vi "GetOutput.vi"(4 "error in":errorcluster, 5 "connection ID":refnum<k5>) -> (0 "Output":string, 1 "error out":errorcluster, 2 "connection ID out":refnum<k5>, 3 "Answer":bool)   [LabVIEW 2013]
panel:
  out "читаю hex":string
  out "читаю текст":string
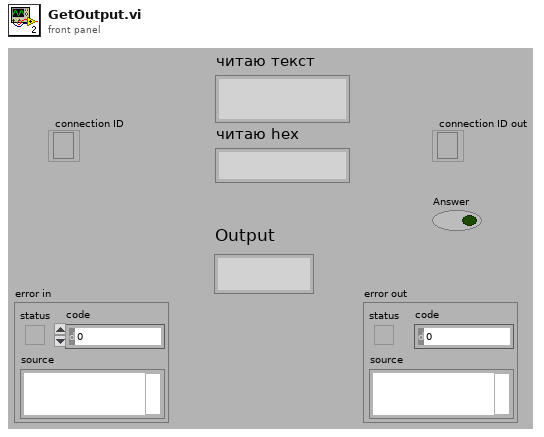
[diagram p1: front panel]
types:
  T1 = enum16{"Standard", "Buffered", "CRLF", "Immediate"}
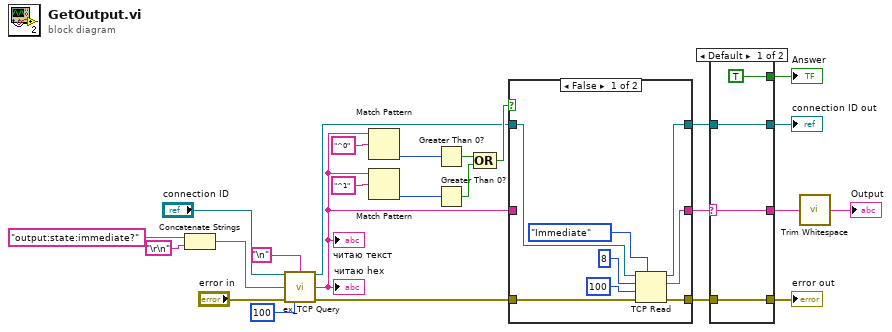
[diagram p0: block diagram]
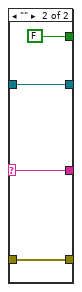
[diagram p3: hidden frame]
diagram:
  n1 = Concatenate Strings("output:state:immediate?" ("data in"), "\r\n") -> (w2:string)
  n2 = call "ex_TCP Query.vi"("TCP Network Connection in"="connection ID", "Termination character"="\n", "Query string"=w2, "error in (no error)"="error in", "Initial byte timeout ms (1000)"=100) -> ("TCP Network Connection out"=w4:refnum<k5>, "Message data out"=w5:string, "error out"=w6:errorcluster)  [unwired: 7 in, 1 out]
  "читаю текст" <- w5
  "читаю hex" <- w5
  n3 = Match Pattern(string=w5, regular expression="^0") -> (offset past match=w19:i32)  [unwired: 1 in, 3 out]
  n4 = Match Pattern(string=w5, regular expression="^1") -> (offset past match=w21:i32)  [unwired: 1 in, 3 out]
  n5 = Greater Than 0?(x=w19) -> (x > 0?=w14:bool)
  n6 = Greater Than 0?(x=w21) -> (x > 0?=w13:bool)
  n7 = Compound Arithmetic op=OR(w14, w13) -> (w12:bool)
  n8 = case shown="False" w12 {
    tunnel: [w27 w36] -> w11
    tunnel: w4 -> [w26 w36]
    tunnel: w6 -> [w30 w35]
    tunnel: [w29 w35] -> w10
    tunnel: w5 -> [_ w34]
    tunnel: [w28 w34] -> w9
    frame False {
      n9 = TCP Read(connection ID=w26, bytes to read=8, error in (no error)=w30, 7:T1."Immediate" ("mode (standard)"), 9:100 ("timeout ms (25000)")) -> (connection ID out=w27:refnum<k5>, data out=w28:string, error out=w29:errorcluster)
    }
    frame True {
    }
  }
  n10 = case shown="Default" w9 {
    selector: w9 -> [w40 w44]
    tunnel: [w40 w44] -> w23
    tunnel: [TRUE FALSE] -> w15
    tunnel: w10 -> [w38 w42]
    tunnel: [w38 w42] -> w17
    tunnel: w11 -> [w37 w41]
    tunnel: [w37 w41] -> w16
    frame Default {
    }
    frame "" {
    }
  }
  "Answer" <- w15
  "connection ID out" <- w16
  "error out" <- w17
  n11 = call <vilib>:"Trim Whitespace.vi"("string"=w23) -> ("trimmed string"=→"Output":string)  [unwired: 1 in]
